vi "Build Transmit Command.vi"(7 "Virtual Memory Unit in":refnum<class "Virtual Memory Unit.lvclass">, 8 "error in (no error)":errorcluster, 10 "Starting Address":u16 format="%04x", 11 "RT-RT Message in":refnum<class "RT-RT Message.lvclass">) -> (0 "error out":errorcluster, 2 "Next Available Address":u16 format="%04x", 3 "RT-RT Message out":refnum<class "RT-RT Message.lvclass">, 5 "Virtual Memory Unit out":refnum<class "Virtual Memory Unit.lvclass">)   [LabVIEW 2020, in "BCI-1553 API.lvlib" / "RT-RT Message.lvclass"]
doc: "Sets up the tx msg command word. This is the 1553 protocol word will be transmittted shortly after the rx cmd word, kicking off the RT-RT transaction."
uses:
  RT-RT Message.lvclass
  Dependencies/Virtual Memory Unit/Virtual Memory Unit.lvclass
  TypeDefs/Command Type.ctl
  RT-RT Message.lvclass/RT-RT Message.ctl
  BCI-1553 API.lvlib
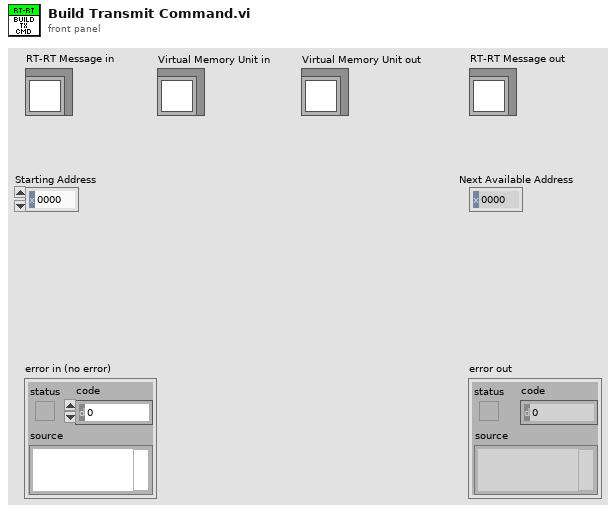
[diagram p1: front panel]
types:
  T1 = typedef "BCI-1553 API.lvlib/Command Type.ctl" = enum16{"Transmit", "Receive"}
  T2 = typedef "BCI-1553 API.lvlib/Command SubAddress.ctl" = enum16{"Mode Code", "1", "2", "3", "4", "5", "6", "7", "8", "9", "10", "11", "12", "13", "14", "15", "16", "17", "18", "19", "20", "21", "22", "23", "24", "25", "26", "27", "28", "29", "30"}
  T3 = typedef "BCI-1553 API.lvlib/Command Word Count.ctl" = enum16{"1", "2", "3", "4", "5", "6", "7", "8", "9", "10", "11", "12", "13", "14", "15", "16", "17", "18", "19", "20", "21", "22", "23", "24", "25", "26", "27", "28", "29", "30", "31", "32"}
  T4 = typedef "BCI-1553 API.lvlib/Command Terminal Address.ctl" = enum16{"0", "1", "2", "3", "4", "5", "6", "7", "8", "9", "10", "11", "12", "13", "14", "15", "16", "17", "18", "19", "20", "21", "22", "23", "24", "25", "26", "27", "28", "29", "30", "Broadcast"}
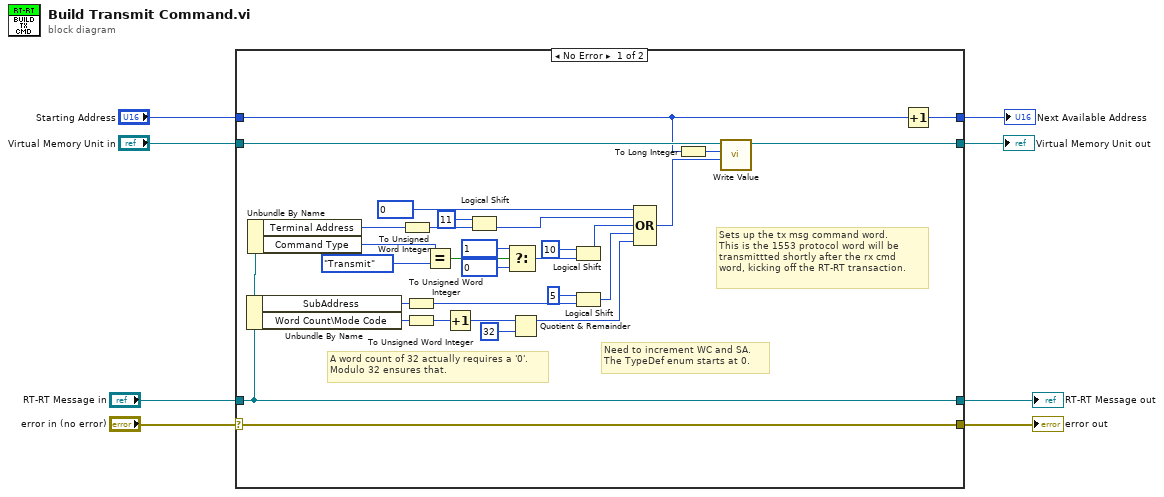
[diagram p0: block diagram]
diagram:
  n1 = case shown="No Error" "error in (no error)" {
    selector: "error in (no error)" -> [w14 w42]
    tunnel: [w14 w42] -> w5
    tunnel: [w32 w41] -> w4
    tunnel: "RT-RT Message in" -> [w32 w41]
    tunnel: "Starting Address" -> [w16 w40]
    tunnel: "Virtual Memory Unit in" -> [w19 w39]
    tunnel: [w18 w39] -> w2
    tunnel: [w38 w40] -> w1
    frame No Error {
      # "Need to increment WC and SA.\nThe TypeDef enum starts at 0."
      # "Sets up the tx msg command word.\nThis is the 1553 protocol word will be\ntransmittted shortly after the rx cmd\nword, kicking off the RT-RT transaction."
      # "A word count of 32 actually requires a '0'.\nModulo 32 ensures that."
      n2 = Unbundle By Name(w32) -> ("SubAddress"=w24:T2, "Word Count\\Mode Code"=w20:T3)
      n3 = Unbundle By Name(w32) -> ("Terminal Address"=w36:T4, "Command Type"=w31:T1)
      n4 = To Unsigned Word Integer(number=w36) -> (unsigned 16bit integer=w13:u16)
      n5 = To Unsigned Word Integer(number=w24) -> (unsigned 16bit integer=w9:u16)
      n6 = To Unsigned Word Integer(number=w20) -> (unsigned 16bit integer=w11:u16)
      n7 = Equal?(x=w31, y=Command_Type."Transmit") -> (x = y?=w30:bool)
      n8 = Increment(x=w11) -> (x+1=w10:u16)
      n9 = Logical Shift(y=i16 11, x=w13) -> (x << y=w35:u16)
      n10 = Select(t=u16 1, s=w30, f=u16 0) -> (s? t:f=w27:u16)
      n11 = Quotient & Remainder(x=w10, y=u16 32) -> (x-y*floor(x/y)=w22:u16)  [unwired: 1 out]
      n12 = Logical Shift(y=i16 10, x=w27) -> (x << y=w26:u16)
      n13 = Logical Shift(y=i16 5, x=w9) -> (x << y=w23:u16)
      n14 = Compound Arithmetic op=OR(u16 0, w35, w26, w23, w22) -> (w17:u16)
      n15 = To Long Integer(number=w16) -> (32bit integer=w15:i32)
      n16 = call "Write Value.vi"("Value"=w17, "Index"=w15, "Virtual Memory Unit in"=w19) -> ("Virtual Memory Unit out"=w18:refnum<class "Virtual Memory Unit.lvclass">)  [unwired: 7 in, 1 out]
      n17 = Increment(x=w16) -> (x+1=w38:u16)
    }
    frame Error {
    }
  }
  "error out" <- w5
  "RT-RT Message out" <- w4
  "Virtual Memory Unit out" <- w2
  "Next Available Address" <- w1
